vi "KepcoDCPwr Revision Query.vi"(0 "VISA Session":refnum<visa-resource-name>, 5 "Model In":string, 7 "channel name (\"\")":string="\"\"", 11 "error in (no error)":errorcluster {"code" format="%.0x"}) -> (4 "VISA Session Out":refnum<visa-resource-name>, 6 "Model Out":string, 8 "channel name out (\"\")":string="\"\"" caption="channel name Out (\"\")", 10 "instrument driver revision":string, 14 "firmware revision":string, 15 "error out":errorcluster {"code" format="%.0x"})   [LabVIEW 2010]
doc: "This VI returns the revision numbers of the instrument firmware."
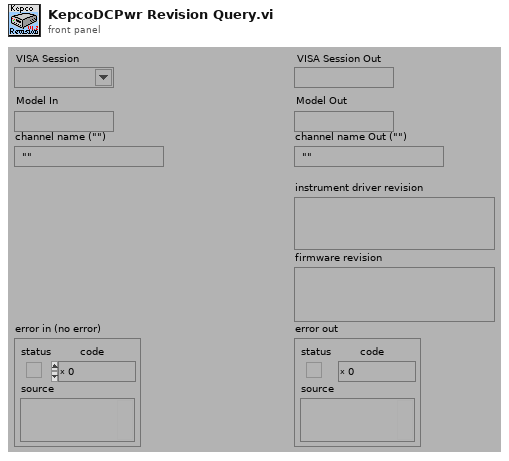
[diagram p1: front panel]
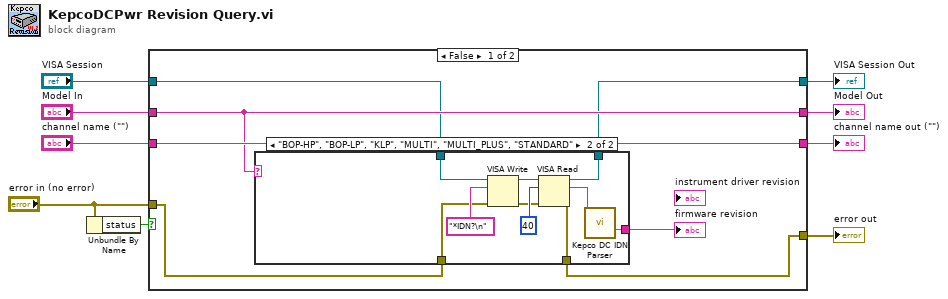
[diagram p0: block diagram]
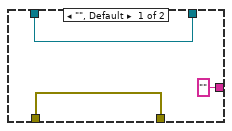
[diagram p2: hidden frame]
diagram:
  n1 = Unbundle By Name("error in (no error)") -> ("status"=w8:bool)
  n2 = case shown="False" w8 {
    tunnel: "error in (no error)" -> [w11 w33]
    tunnel: [w12 w33] -> w7
    tunnel: [w13 w32] -> w3
    tunnel: "VISA Session" -> [w14 w32]
    tunnel: [w15 w31] -> w2
    tunnel: "Model In" -> [w15 w31]
    tunnel: "channel name (\"\")" -> [w16 w30]
    tunnel: [w16 w30] -> w1
    frame False {
      n3 = case shown="\"BOP-HP\", \"BOP-LP\", \"KLP\", \"MULTI\", \"MULTI_PLUS\", \"STANDARD\"" w15 {
        tunnel: w14 -> [w19 w24]
        tunnel: w11 -> [w18 w23]
        tunnel: [w19 w22] -> w13
        tunnel: [w18 w21] -> w12
        tunnel: ["" ("Firmware Version") w20] -> w10
        frame "", Default {
        }
        frame "BOP-HP", "BOP-LP", "KLP", "MULTI", "MULTI_PLUS", "STANDARD" {
          n4 = VISA Write(VISA resource name=w24, write buffer="*IDN?\n" ("write buffer (\"\")"), error in (no error)=w23) -> (VISA resource name out=w29:refnum<visa-resource-name>, error out=w25:errorcluster)  [unwired: 1 out]
          n5 = VISA Read(VISA resource name=w29, byte count=u32 40 ("byte count (0)"), error in (no error)=w25) -> (VISA resource name out=w22:refnum<visa-resource-name>, read buffer=w27:string, error out=w21:errorcluster)  [unwired: 1 out]
          n6 = call "Kepco DC IDN Parser.vi"("IDN Query"=w27) -> ("Firmware Version"=w20:string)  [unwired: 9 in, 5 out]
        }
      }
      "firmware revision" <- w10
    }
    frame True {
    }
  }
  "error out" <- w7
  "channel name out (\"\")" <- w1
  "Model Out" <- w2
  "VISA Session Out" <- w3
